vi "Report.Create.vi"(7 "Result Directory":path, 8 "error in (no error)":errorcluster, 10 "Results":variant, 11 "Data Path":path) -> (0 "error out":errorcluster)   [LabVIEW 2015, in "NIAnalysis.lvlib"]
uses:
  NIAnalysis.lvlib
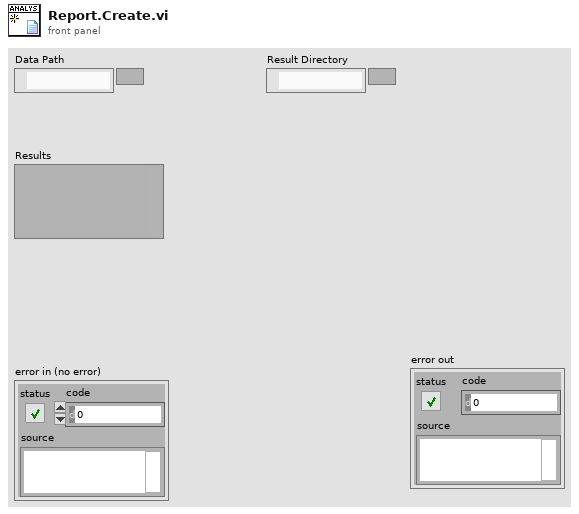
[diagram p1: front panel]
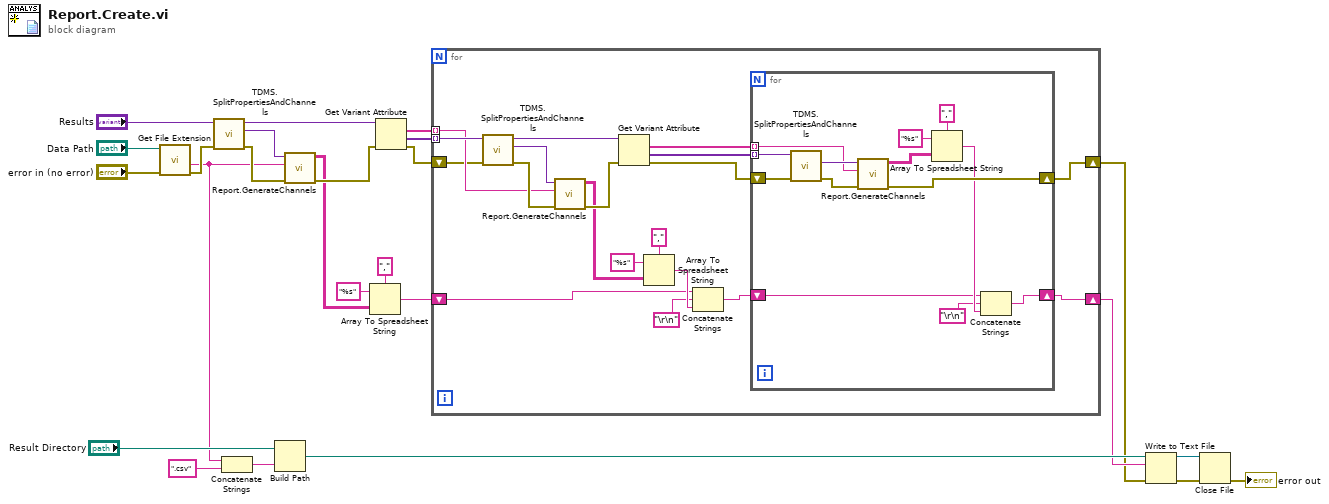
[diagram p0: block diagram]
diagram:
  n1 = call <vilib>:"Get File Extension.vi"("error in (no error)"="error in (no error)", "file"="Data Path") -> ("error out"=w18:errorcluster, "filename without extension"=w9:string)  [unwired: 5 in, 3 out]
  n2 = call "TDMS.SplitPropertiesAndChannels.vi"("error in"=w18, "Properties"="Results") -> ("error out"=w17:errorcluster, "Properties"=w16:variant, "Channels"=w23:variant)  [unwired: 7 in]
  n3 = Concatenate Strings(w9, ".csv" ("string")) -> (w7:string)
  n4 = Build Path(base path="Result Directory", name or relative path=w7) -> (appended path=w6:path)
  n5 = call "Report.GenerateChannels.vi"("error in (no error)"=w17, "Channel"=w9, "Properties"=w16) -> ("error out"=w15:errorcluster, "Reports"=w12:string[][])  [unwired: 7 in]
  n6 = Array To Spreadsheet String(delimiter (Tab)=",", array=w12, 3:"%s" ("format string")) -> (spreadsheet string=w11:string)
  n7 = Get Variant Attribute(Variant=w23, error in=w15) -> (names=w21:string[], values=w20:variant[], error out=w22:errorcluster)  [unwired: 2 in, 1 out]
  n8 = for {
    tunnel: w21 -> [w32] mode=indexing
    tunnel: w20 -> [w41] mode=indexing
    shift-right: [w39] -> w2
    shift-left: w22 -> [w31]
    shift-right: [w27] -> w3
    shift-left: w11 -> [w28]
    n9 = call "TDMS.SplitPropertiesAndChannels.vi"("error in"=w31, "Properties"=w41) -> ("error out"=w37:errorcluster, "Properties"=w38:variant, "Channels"=w40:variant)  [unwired: 7 in]
    n10 = call "Report.GenerateChannels.vi"("error in (no error)"=w37, "Channel"=w32, "Properties"=w38) -> ("error out"=w36:errorcluster, "Reports"=w33:string[][])  [unwired: 7 in]
    n11 = Get Variant Attribute(Variant=w40, error in=w36) -> (names=w44:string[], values=w42:variant[], error out=w43:errorcluster)  [unwired: 2 in, 1 out]
    n12 = Array To Spreadsheet String(delimiter (Tab)=",", array=w33, 3:"%s" ("format string")) -> (spreadsheet string=w30:string)
    n13 = Concatenate Strings(w28, "\r\n", w30) -> (w29:string)
    n14 = for {
      tunnel: w44 -> [w55] mode=indexing
      shift-right: [w52] -> w39
      shift-left: w43 -> [w54]
      tunnel: w42 -> [w57] mode=indexing
      shift-right: [w46] -> w27
      shift-left: w29 -> [w47]
      n15 = call "TDMS.SplitPropertiesAndChannels.vi"("error in"=w54, "Properties"=w57) -> ("error out"=w53:errorcluster, "Properties"=w56:variant)  [unwired: 7 in, 1 out]
      n16 = call "Report.GenerateChannels.vi"("error in (no error)"=w53, "Channel"=w55, "Properties"=w56) -> ("error out"=w52:errorcluster, "Reports"=w51:string[][])  [unwired: 7 in]
      n17 = Array To Spreadsheet String(delimiter (Tab)=",", array=w51, 3:"%s" ("format string")) -> (spreadsheet string=w48:string)
      n18 = Concatenate Strings(w47, "\r\n", w48) -> (w46:string)
    }
  }
  n19 = Write to Text File(file (use dialog)=w6, text=w3, error in=w2) -> (refnum out=w4:refnum<file>, error out=w5:errorcluster)  [unwired: 1 in, 1 out]
  n20 = Close File(refnum=w4, error in=w5) -> (error out=→"error out":errorcluster)  [unwired: 1 out]
